vi "getSkipMessage.vi"(8 "error in (no error)":errorcluster, 11 "TestCase in":refnum<class "TestCase.lvclass">) -> (0 "error out":errorcluster, 2 "skipMessage":string, 3 "TestCase out":refnum<class "TestCase.lvclass">)   [LabVIEW 2011, in "TestCase.lvclass"]
uses:
  TestCase.lvclass
  TestCase.lvclass/TestCase.ctl
panel:
  # "JKI VI Tester for LabVIEW\nhttp://jkisoft.com/vi-tester\nCopyright (C) 2007-2009, JKI <info@jkisoft.com>\nALL RIGHTS RESERVED"
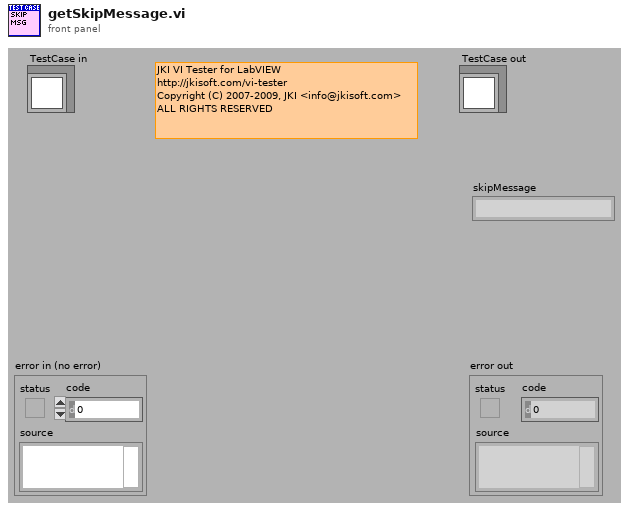
[diagram p1: front panel]
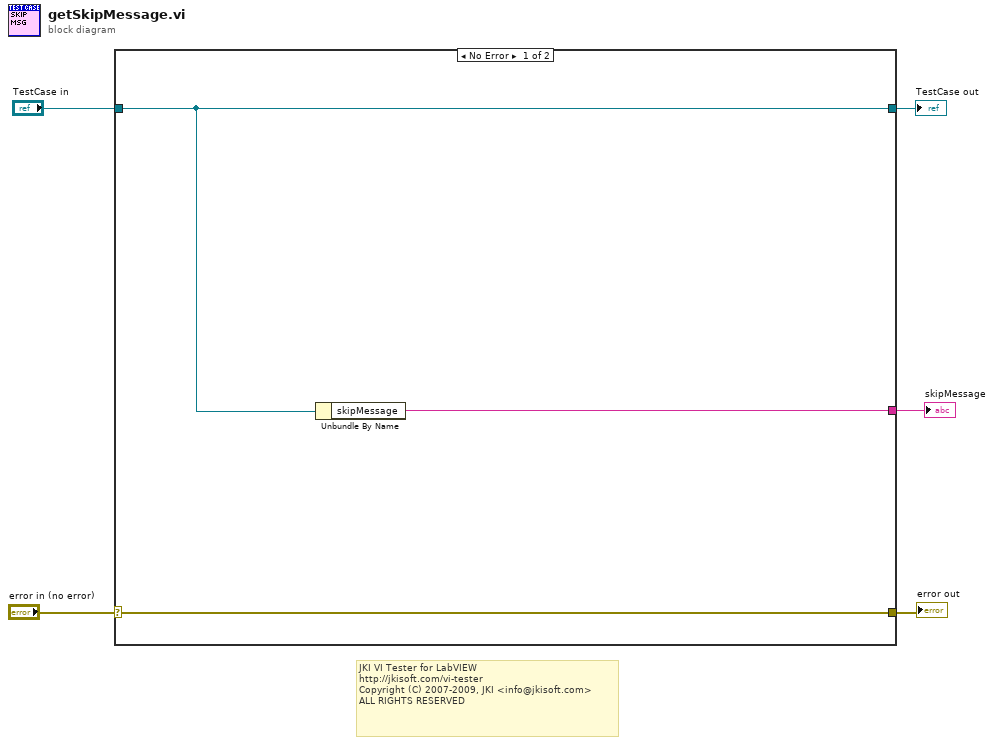
[diagram p0: block diagram]
diagram:
  # "JKI VI Tester for LabVIEW\nhttp://jkisoft.com/vi-tester\nCopyright (C) 2007-2009, JKI <info@jkisoft.com>\nALL RIGHTS RESERVED"
  n1 = case shown="No Error" "error in (no error)" {
    selector: "error in (no error)" -> [w7 w10]
    tunnel: [w7 w10] -> w4
    tunnel: [w8 w9] -> w2
    tunnel: "TestCase in" -> [w8 w9]
    tunnel: [w6 _] -> w1
    frame No Error {
      n2 = Unbundle By Name(w8) -> ("skipMessage"=w6:string)
    }
    frame Error {
    }
  }
  "error out" <- w4
  "TestCase out" <- w2
  "skipMessage" <- w1
